vi "Convert from Degrees C per Second.vi"(4 "Rate In":dbl, 5 "Rate Units":T2, 6 "Temp Units":T1) -> (7 "Rate Out":dbl)   [LabVIEW 2024, in "_Thermal Process Controller.lvclass"]
uses:
  _Thermal Process Controller.lvclass
  Controls/Rate Units--Enum.ctl
  Controls/Temperature Units--Enum.ctl
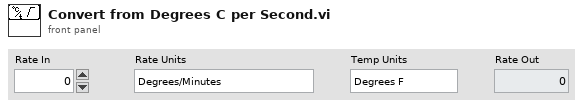
[diagram p1: front panel]
types:
  T1 = typedef "_Thermal Process Controller.lvclass/Temperature Units--Enum.ctl" = enum16{"Degrees F", "Degrees C", "Degrees K"}
  T2 = typedef "_Thermal Process Controller.lvclass/Rate Units--Enum.ctl" = enum16{"Degrees/Minutes", "Degrees/Hours"}
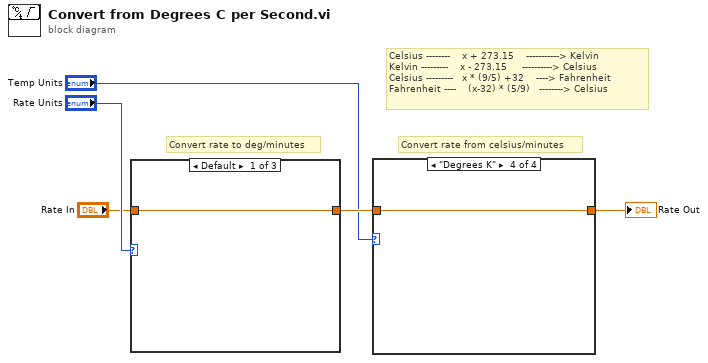
[diagram p0: block diagram]
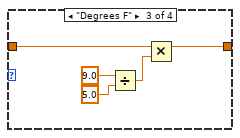
[diagram p4: hidden frame]
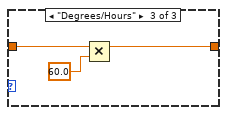
[diagram p6: hidden frame]
diagram:
  # "Celsius --------    x + 273.15    -----------> Kelvin\nKelvin ---------    x - 273.15     ----------> Celsius\nCelsius ---------   x * (9/5) +32    ----> Fahrenheit\nFahrenheit ----    (x-32) * (5/9)   --------> Celsius"
  # "Convert rate from celsius/minutes"
  # "Convert rate to deg/minutes"
  n1 = case shown="Default" "Rate Units" {
    tunnel: [w6 w7 w9] -> w3
    tunnel: "Rate In" -> [w6 w7 w10]
    frame Default {
    }
    frame "Degrees/Minutes" {
    }
    frame "Degrees/Hours" {
      n2 = Multiply(x=w10, y=60.0) -> (x*y=w9:dbl)
    }
  }
  n3 = case shown="\"Degrees K\"" "Temp Units" {
    tunnel: w3 -> [w11 w12 w15 w18]
    tunnel: [w11 w12 w13 w18] -> w1
    frame Default {
    }
    frame "Degrees C" {
    }
    frame "Degrees F" {
      n4 = Divide(x=9.0, y=5.0) -> (x/y=w14:dbl)
      n5 = Multiply(x=w15, y=w14) -> (x*y=w13:dbl)
    }
    frame "Degrees K" {
    }
  }
  "Rate Out" <- w1
